vi "Teleop.vi"(10 "Match Info":T1={"Autonomous Elapsed Seconds"=0.0, "TeleOp Elapsed Seconds"=0.0, "Disabled Elapsed Seconds"=0.0, "Visited Autonomous"=FALSE, "Visited TeleOp"=FALSE, "Visited Disabled"=FALSE, "Autonomous Settings"={"Autonomous Style"=enum."Independent", "VI Refnum"=refnum}}, 11 "Call Context":T2) -> ()   [LabVIEW 2012]
doc: "This VI is called for each TeleOp packet received from the DS where the robot is not disabled. It is often used to read from the joysticks and update I/O or to update setpoints for timed control loops. It should complete and return within 20 milliseconds or it may miss DS packets."
uses:
  <vilib>/Rock Robotics/WPI/DriverStation/WPI_DriverStationDerivedRobotMode.ctl
  <vilib>/Rock Robotics/WPI/DriverStation/WPI_DriverStationMatch Info.ctl
  <vilib>/Rock Robotics/WPI/Joystick/WPI_JoystickAxis.ctl
  <vilib>/Rock Robotics/WPI/DriverStation/DriverStationLCD/WPI_DriverStationLCDLCDLine.ctl
  <vilib>/Rock Robotics/WPI/Solenoid/WPI_SolenoidValue.ctl
  Robot Global Data.vi
  <vilib>/Rock Robotics/WPI/Joystick/WPI_JoystickGetSetRefNum.vi
  <vilib>/Rock Robotics/WPI/RobotDrive/WPI_RobotDriveGetSetRefNum.vi
  <vilib>/Rock Robotics/WPI/Solenoid/WPI_SolenoidSetEnum.vi
panel:
  in  "ShifterState":bool
  in  "LifterState":bool
  out "Numeric 1":dbl(slide) scale=0.0..100.0
  out "Boolean 2":bool
  out "Boolean 1":bool
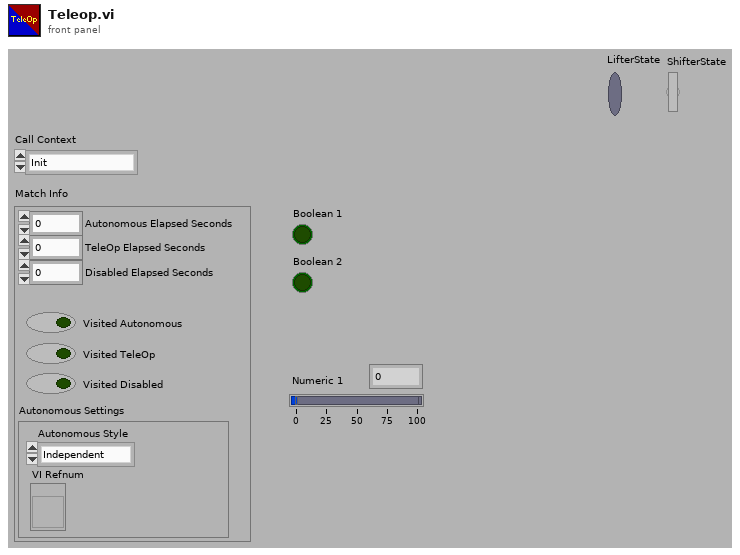
[diagram p1: front panel]
types:
  T1 = typedef "WPI_DriverStationMatch Info.ctl" = cluster{"Autonomous Elapsed Seconds":dbl, "TeleOp Elapsed Seconds":dbl, "Disabled Elapsed Seconds":dbl, "Visited Autonomous":bool, "Visited TeleOp":bool, "Visited Disabled":bool, "Autonomous Settings":cluster{"Autonomous Style":enum16{"Iterative", "Independent"}, "VI Refnum":refnum<vi>}}
  T2 = typedef "WPI_DriverStationDerivedRobotMode.ctl" = enum16{"Init", "Execute", "Stop"}
  T3 = typedef "WPI_JoystickAxis.ctl" = enum16{"Axis 1", "Axis 2", "Axis 3", "Axis 4", "Axis 5", "Axis 6"}
  T4 = typedef "WPI_JoystickDevRef.ctl" = cluster{"Device":T5}
  T5 = typedef "WPI_JoystickDeviceEnum.ctl" = enum16{"USB 1", "USB 2", "USB 3", "USB 4", "Kinect 1", "Kinect 2"}
  T6 = typedef "WPI_JoystickButtonState.ctl" = cluster{"Button 1":bool, "Button 2":bool, "Button 3":bool, "Button 4":bool, "Button 5":bool, "Button 6":bool, "Button 7":bool, "Button 8":bool, "Button 9":bool, "Button 10":bool, "Button 11":bool, "Button 12":bool}
  T7 = cluster{"axis 1 (x)":dbl, "axis 2 (y)":dbl, "axis 3 (throttle)":dbl, "axis 4":dbl, "axis 5":dbl, "axis 6":dbl}
  T8 = typedef "WPI_DriverStationLCDLCDLine.ctl" = enum16{"Main - Line 1", "User - Line 2", "User - Line 3", "User - Line 4", "User - Line 5", "User - Line 6"}
  T9 = typedef "WPI_SolenoidValue.ctl" = enum16{"Off", "On", "Forward", "Reverse"}
  T10 = typedef "WPI_MotorControlDeviceRef.ctl" = cluster{"DeviceStatus":errorcluster, "Type":enum16{"PWM", "CAN"}, "PWM":cluster{"Digital Module":T11, "PWM Channel":T12, "DeadBand":T13}, "CAN":cluster{"Device Number":u8, "Control Mode":T14, "Semaphore":T15, "Max Vout":dbl}, "Invert":bool, "TransformRef":T16, "InvTransformRef":T16}
  T11 = typedef "FPGA_TypedefDigitalModule.ctl" = enum16{"Digital Module 1", "Digital Module 2"}
  T12 = typedef "FPGA_DIOPWMChannel.ctl" = enum8{"PWM 1", "PWM 2", "PWM 3", "PWM 4", "PWM 5", "PWM 6", "PWM 7", "PWM 8", "PWM 9", "PWM 10", "Invalid"}
  T13 = typedef "WPI_PWMDeadband.ctl" = cluster{"Name":string, "maxPositivePwm":i32, "minPositivePwm":i32, "centerPwm":i32, "maxNegativePwm":i32, "minNegativePwm":i32, "angularRange":u16}
  T14 = typedef "WPI_CANJaguar_ControlMode.ctl" = enum8{"Percent VBus", "Current", "Speed", "Position", "Voltage"}
  T15 = typedef "Semaphore RefNum" = refnum<k1>
  T16 = typedef "WPI_PWMTransform_ConPane.ctl" = refnum<vi>
  T17 = typedef "WPI_SolenoidDevRef.ctl" = cluster{"DevStatus":errorcluster, "Solenoid Module":T18, "Forward Solenoid Channel":T19, "Reverse Solenoid Channel":T19}
  T18 = typedef "FPGA_TypedefSolenoidModule.ctl" = enum16{"Solenoid Module 1", "Solenoid Module 2"}
  T19 = typedef "WPI_SolenoidChannel.ctl" = enum8{"Solenoid 1", "Solenoid 2", "Solenoid 3", "Solenoid 4", "Solenoid 5", "Solenoid 6", "Solenoid 7", "Solenoid 8", "Invalid"}
  T20 = typedef "WPI_RobotDriveDevRef.ctl" = cluster{"DevStatus":errorcluster, "Motors[]":T10[], "Square Inputs":bool, "Max Output":dbl, "Isochronous":bool}
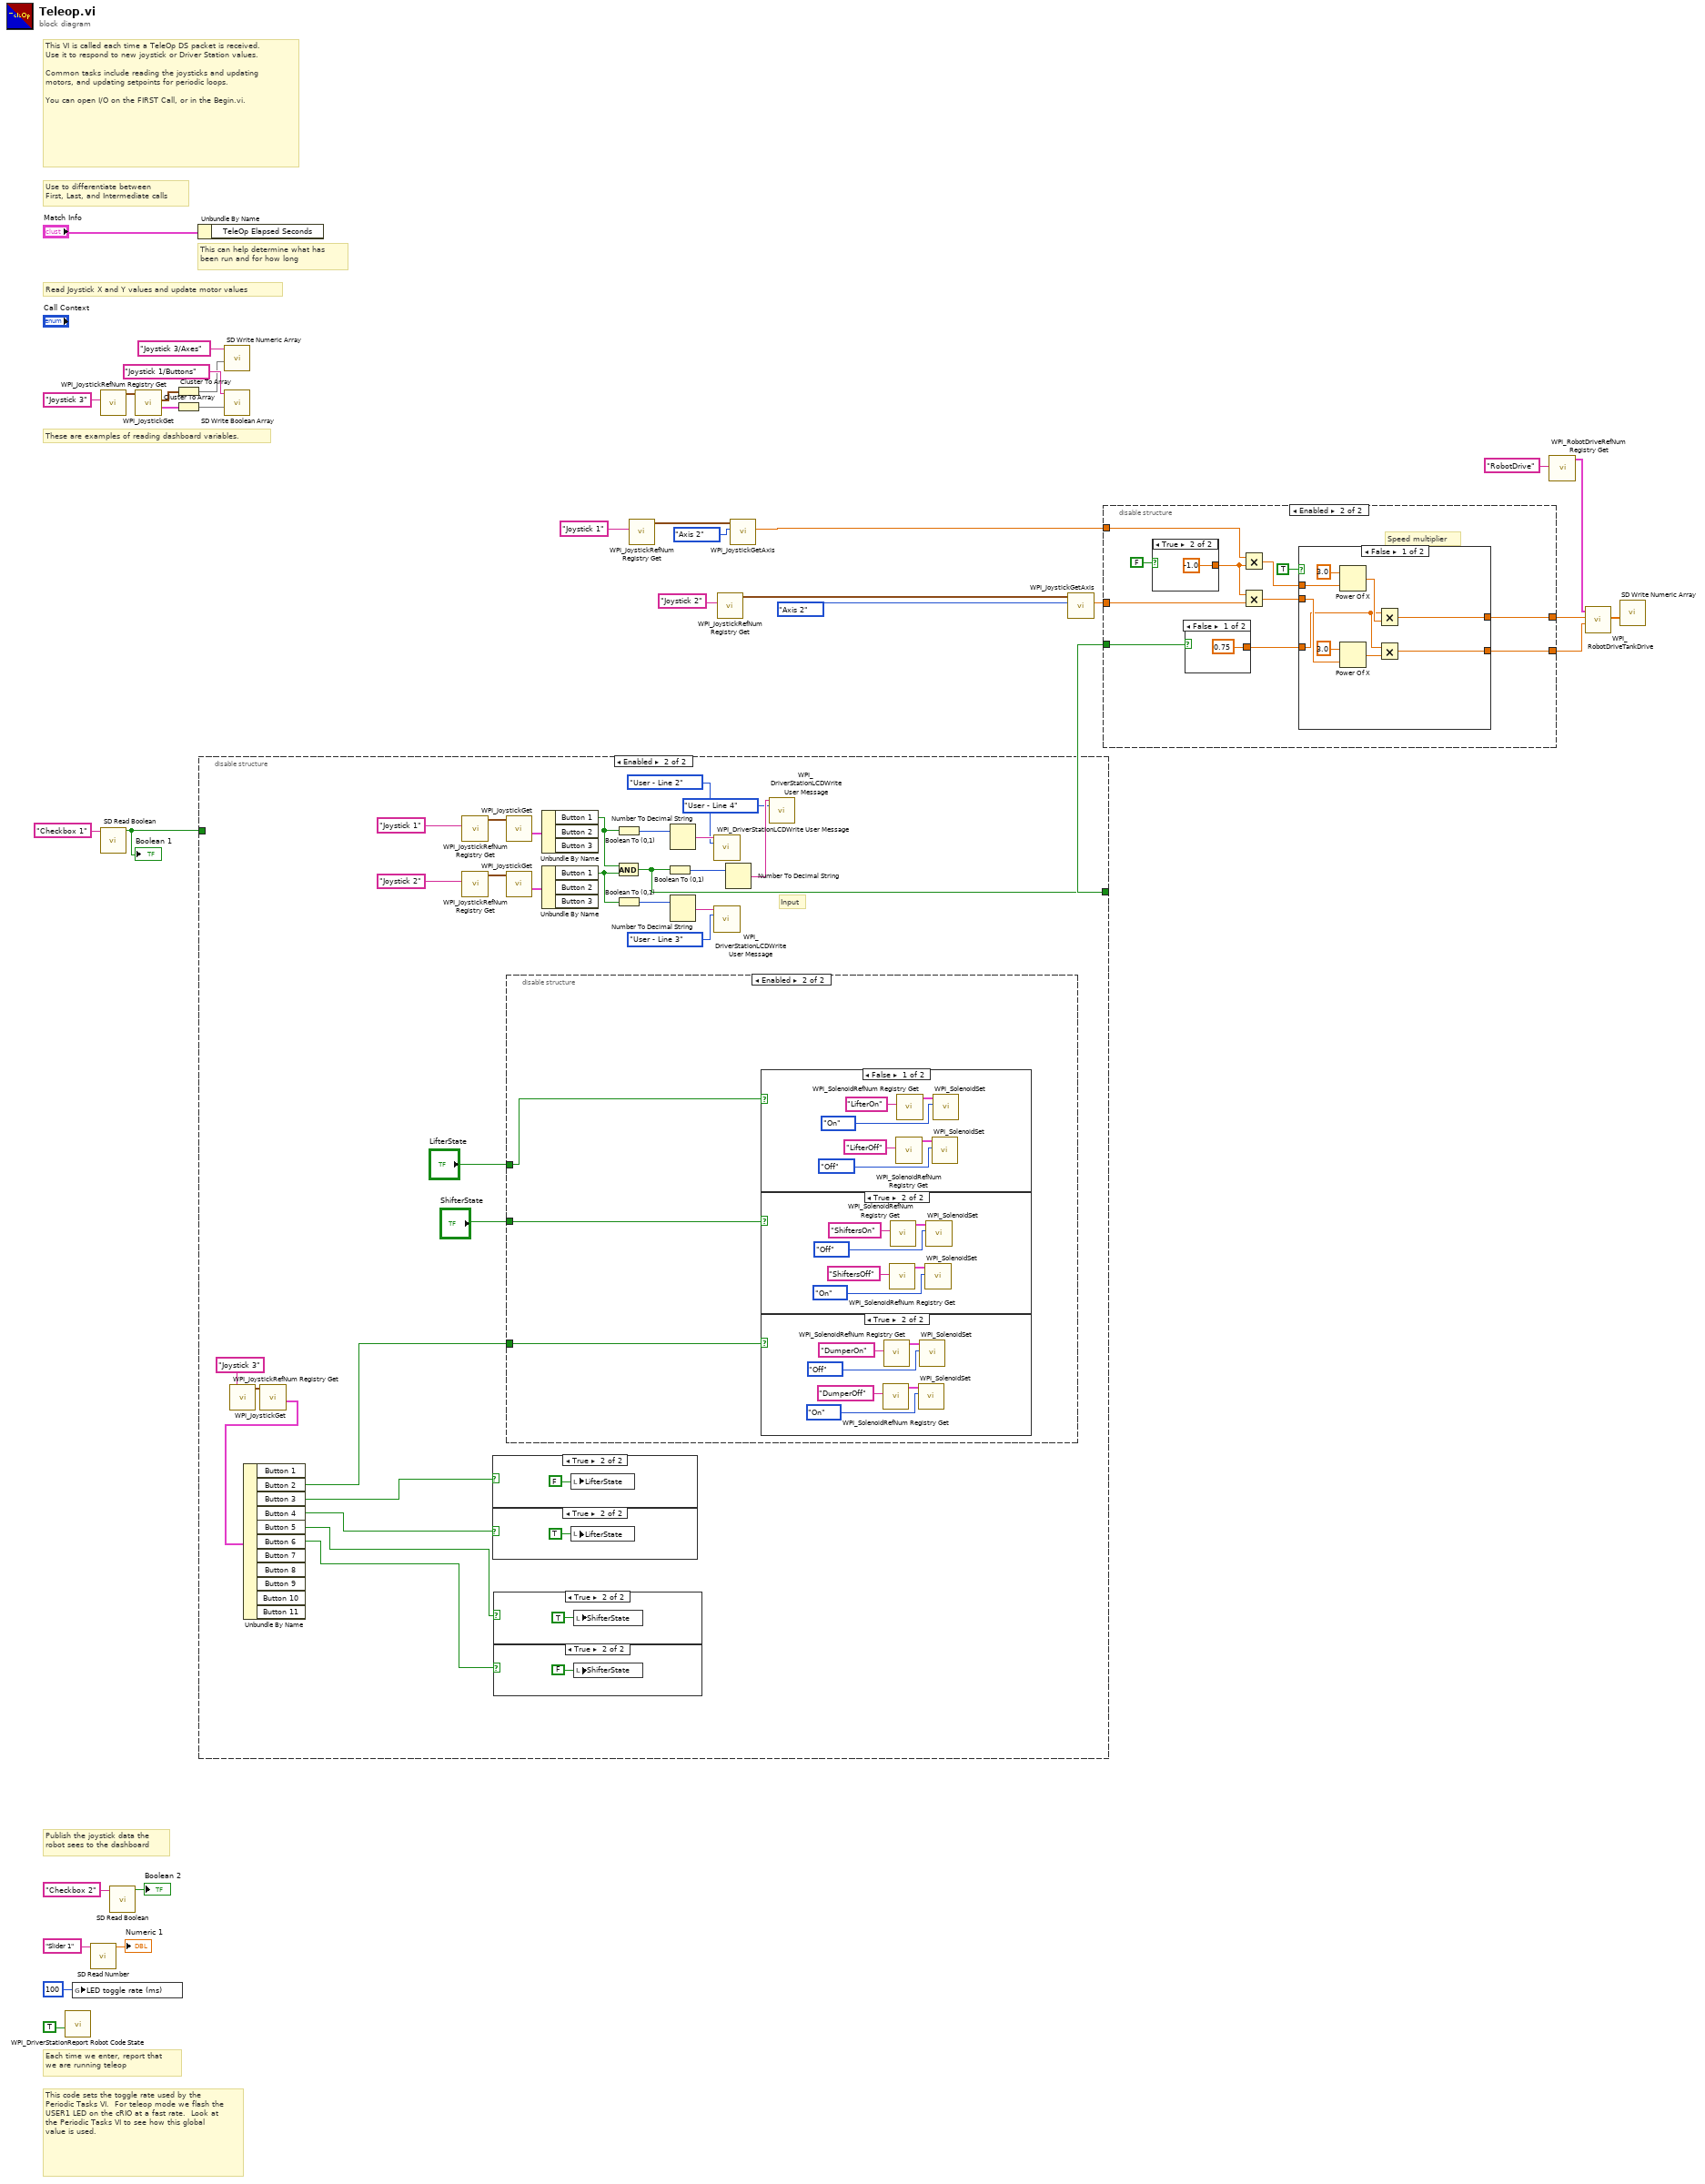
[diagram p0: block diagram]
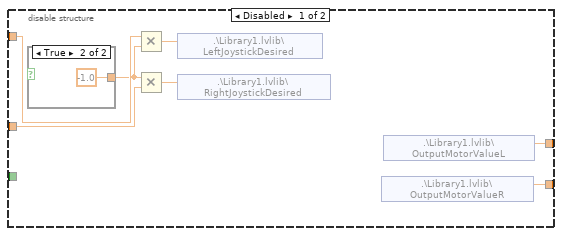
[diagram p2: hidden frame]
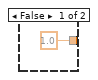
[diagram p3: hidden frame]
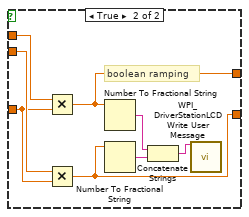
[diagram p4: hidden frame]
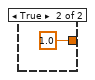
[diagram p5: hidden frame]
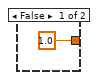
[diagram p6: hidden frame]
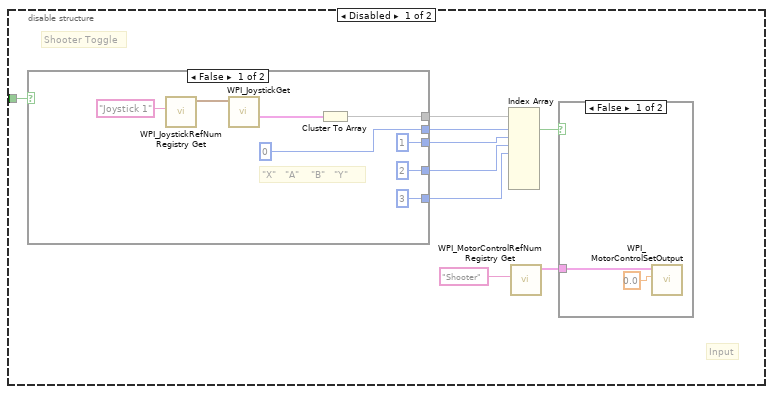
[diagram p7: hidden frame]
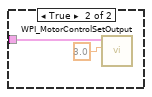
[diagram p8: hidden frame]
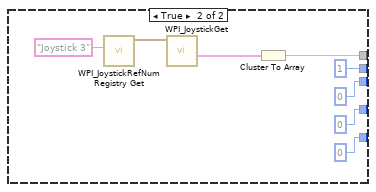
[diagram p9: hidden frame]
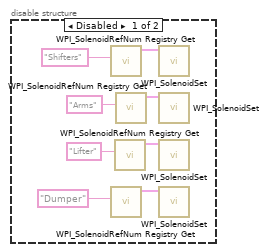
[diagram p14: hidden frame]
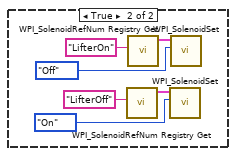
[diagram p15: hidden frame]
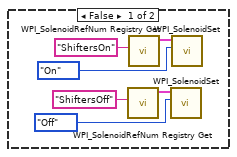
[diagram p16: hidden frame]
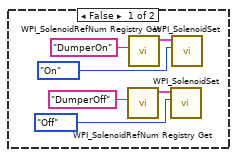
[diagram p17: hidden frame]
diagram:
  # "This code sets the toggle rate used by the Periodic Tasks VI.  For teleop mode we flash the USER1 LED on the cRIO at a fast rate.  Look at the Periodic Tasks VI to see how this global value is used."
  # "This VI is called each time a TeleOp DS packet is received.  Use it to respond to new joystick or Driver Station values.\n\nCommon tasks include reading the joysticks and updating motors, and updating setpoints for periodic loops.\n\nYou can open I/O on the FIRST Call, or in the Begin.vi."
  # "Publish the joystick data the\nrobot sees to the dashboard"
  # "These are examples of reading dashboard variables."
  # "Each time we enter, report that\nwe are running teleop"
  # "Use to differentiate between\nFirst, Last, and Intermediate calls"
  # "This can help determine what has\nbeen run and for how long"
  # "Read Joystick X and Y values and update motor values"
  n1 = call <vilib>:"WPI_DriverStationReport Robot Code State.vi"("TeleOp"=TRUE ("Autonomous")) -> ()  [unwired: 10 in, 1 out]
  n2 = global write "Robot Global Data.vi" "LED toggle rate (ms)"(u32 100 ("LED ms toggle rate")) -> ()
  n3 = call <vilib>:"SD Read Number.vi"("Name"="Slider 1" ("refnum name")) -> ("Numeric"=→"Numeric 1":dbl)  [unwired: 8 in, 2 out]
  n4 = call <vilib>:"WPI_JoystickRefNum Registry Get.vi"("refnum name"="Joystick 3") -> ("JoystickDevRef"=w22:T4)  [unwired: 1 in, 9 out]
  n5 = call <vilib>:"SD Read Boolean.vi"("Name"="Checkbox 1" ("refnum name")) -> ("Boolean"=w9:bool)  [unwired: 8 in, 2 out]
  "Boolean 1" <- w9
  n6 = call <vilib>:"SD Read Boolean.vi"("Name"="Checkbox 2" ("refnum name")) -> ("Boolean"=→"Boolean 2":bool)  [unwired: 8 in, 2 out]
  n7 = call <vilib>:"WPI_JoystickGet.vi"("JoystickDevRef"=w22) -> ("Buttons"=w21:T6, "Axes"=w18:T7)  [unwired: 1 in, 4 out]
  n8 = Cluster To Array(cluster=w18) -> (array=w20:dbl[])
  n9 = Cluster To Array(cluster=w21) -> (array=w25:bool[])
  n10 = Unbundle By Name("Match Info") -> ()  [unwired: 1 out]
  n11 = disable-structure shown="Enabled" {
    disable-tunnel: w9 -> [w40 _]
    disable-tunnel: [_ w74] -> w2
    frame Disabled {
      # "Input"
      # "Shooter Toggle"
      n12 = case shown="False" w40 {
        tunnel: [0 ("index") 1 ("index")] -> w39
        tunnel: [1 ("index") 0 ("index")] -> w34
        tunnel: [2 ("index") 0 ("index")] -> w36
        tunnel: [3 ("index") 0 ("index")] -> w35
        tunnel: [w48 w60] -> w37
        frame False {
          # "\"X\"   \"A\"    \"B\"   \"Y\""
          n13 = call <vilib>:"WPI_JoystickRefNum Registry Get.vi"("refnum name"="Joystick 1") -> ("JoystickDevRef"=w46:T4)  [unwired: 9 in, 1 out]
          n14 = call <vilib>:"WPI_JoystickGet.vi"("JoystickDevRef"=w46) -> ("Buttons"=w47:T6)  [unwired: 4 in, 2 out]
          n15 = Cluster To Array(cluster=w47) -> (array=w48:bool[])
        }
        frame True {
          n16 = call <vilib>:"WPI_JoystickRefNum Registry Get.vi"("refnum name"="Joystick 3") -> ("JoystickDevRef"=w58:T4)  [unwired: 9 in, 1 out]
          n17 = call <vilib>:"WPI_JoystickGet.vi"("JoystickDevRef"=w58) -> ("Buttons"=w59:T6)  [unwired: 4 in, 2 out]
          n18 = Cluster To Array(cluster=w59) -> (array=w60:bool[])
        }
      }
      n19 = Index Array(array=w37, index #1=w39, index #2=w34, index #3=w36, index #4=w35) -> (element #1=w38:bool)  [unwired: 4 in, 7 out]
      n20 = call <vilib>:"WPI_MotorControlRefNum Registry Get.vi"("refnum name"="Shooter") -> ("MotorControlDevRef"=w33:T10)  [unwired: 9 in, 1 out]
      n21 = case shown="False" w38 {
        tunnel: w33 -> [w42 w44]
        frame False {
          n22 = call <vilib>:"WPI_MotorControlSetOutput.vi"("Output"=0.0, "MotorControlDevRef"=w42) -> ()  [unwired: 7 in, 3 out]
        }
        frame True {
          n23 = call <vilib>:"WPI_MotorControlSetOutput.vi"("Output"=3.0, "MotorControlDevRef"=w44) -> ()  [unwired: 7 in, 3 out]
        }
      }
    }
    frame Enabled {
      # "Input"
      n24 = call <vilib>:"WPI_JoystickRefNum Registry Get.vi"("refnum name"="Joystick 3") -> ("JoystickDevRef"=w86:T4)  [unwired: 9 in, 1 out]
      n25 = call <vilib>:"WPI_JoystickGet.vi"("JoystickDevRef"=w86) -> ("Buttons"=w81:T6)  [unwired: 4 in, 2 out]
      n26 = Unbundle By Name(w81) -> ("Button 2"=w65:bool, "Button 3"=w64:bool, "Button 4"=w63:bool, "Button 5"=w62:bool, "Button 6"=w61:bool)  [unwired: 6 out]
      n27 = call <vilib>:"WPI_JoystickRefNum Registry Get.vi"("refnum name"="Joystick 1") -> ("JoystickDevRef"=w84:T4)  [unwired: 9 in, 1 out]
      n28 = call <vilib>:"WPI_JoystickRefNum Registry Get.vi"("refnum name"="Joystick 2") -> ("JoystickDevRef"=w80:T4)  [unwired: 9 in, 1 out]
      n29 = case shown="True" w64 {
        frame False {
        }
        frame True {
          n30 = local write "LifterState"(FALSE ("ArmState")) -> ()
        }
      }
      n31 = case shown="True" w63 {
        frame False {
        }
        frame True {
          n32 = local write "LifterState"(TRUE ("ArmState")) -> ()
        }
      }
      n33 = case shown="True" w62 {
        frame False {
        }
        frame True {
          n34 = local write "ShifterState"(TRUE ("ArmState")) -> ()
        }
      }
      n35 = case shown="True" w61 {
        frame False {
        }
        frame True {
          n36 = local write "ShifterState"(FALSE ("ArmState")) -> ()
        }
      }
      n37 = call <vilib>:"WPI_JoystickGet.vi"("JoystickDevRef"=w84) -> ("Buttons"=w82:T6)  [unwired: 4 in, 2 out]
      n38 = call <vilib>:"WPI_JoystickGet.vi"("JoystickDevRef"=w80) -> ("Buttons"=w78:T6)  [unwired: 4 in, 2 out]
      n39 = disable-structure shown="Enabled" {
        disable-tunnel: "LifterState" -> [_ w102]
        disable-tunnel: "ShifterState" -> [_ w103]
        disable-tunnel: w65 -> [_ w101]
        frame Disabled {
          n40 = call <vilib>:"WPI_SolenoidRefNum Registry Get.vi"("refnum name"="Shifters") -> ("SolenoidDevRef"=w99:T17)  [unwired: 9 in, 1 out]
          n41 = call <vilib>:"WPI_SolenoidRefNum Registry Get.vi"("refnum name"="Dumper") -> ("SolenoidDevRef"=w94:T17)  [unwired: 9 in, 1 out]
          n42 = call <vilib>:"WPI_SolenoidRefNum Registry Get.vi"("refnum name"="Lifter") -> ("SolenoidDevRef"=w98:T17)  [unwired: 9 in, 1 out]
          n43 = call <vilib>:"WPI_SolenoidRefNum Registry Get.vi"("refnum name"="Arms") -> ("SolenoidDevRef"=w96:T17)  [unwired: 9 in, 1 out]
          n44 = call-poly <vilib>:"WPI_SolenoidSet.vi"("SolenoidDevRef"=w99) -> ()  [unwired: 9 in, 2 out]
          n45 = call-poly <vilib>:"WPI_SolenoidSet.vi"("SolenoidDevRef"=w96) -> ()  [unwired: 9 in, 2 out]
          n46 = call-poly <vilib>:"WPI_SolenoidSet.vi"("SolenoidDevRef"=w98) -> ()  [unwired: 9 in, 2 out]
          n47 = call-poly <vilib>:"WPI_SolenoidSet.vi"("SolenoidDevRef"=w94) -> ()  [unwired: 9 in, 2 out]
        }
        frame Enabled {
          n48 = case shown="False" w102 {
            frame False {
              n49 = call <vilib>:"WPI_SolenoidRefNum Registry Get.vi"("refnum name"="LifterOff") -> ("SolenoidDevRef"=w106:T17)  [unwired: 9 in, 1 out]
              n50 = call <vilib>:"WPI_SolenoidRefNum Registry Get.vi"("refnum name"="LifterOn") -> ("SolenoidDevRef"=w108:T17)  [unwired: 9 in, 1 out]
              n51 = call-poly <vilib>:"WPI_SolenoidSet.vi"("Value"=WPI_SolenoidValue."Off", "SolenoidDevRef"=w106) -> ()  [unwired: 8 in, 2 out]
              n52 = call-poly <vilib>:"WPI_SolenoidSet.vi"("Value"=WPI_SolenoidValue."On", "SolenoidDevRef"=w108) -> ()  [unwired: 8 in, 2 out]
            }
            frame True {
              n53 = call <vilib>:"WPI_SolenoidRefNum Registry Get.vi"("refnum name"="LifterOff") -> ("SolenoidDevRef"=w112:T17)  [unwired: 9 in, 1 out]
              n54 = call <vilib>:"WPI_SolenoidRefNum Registry Get.vi"("refnum name"="LifterOn") -> ("SolenoidDevRef"=w114:T17)  [unwired: 9 in, 1 out]
              n55 = call-poly <vilib>:"WPI_SolenoidSet.vi"("Value"=WPI_SolenoidValue."On", "SolenoidDevRef"=w112) -> ()  [unwired: 8 in, 2 out]
              n56 = call-poly <vilib>:"WPI_SolenoidSet.vi"("Value"=WPI_SolenoidValue."Off", "SolenoidDevRef"=w114) -> ()  [unwired: 8 in, 2 out]
            }
          }
          n57 = case shown="True" w103 {
            frame False {
              n58 = call <vilib>:"WPI_SolenoidRefNum Registry Get.vi"("refnum name"="ShiftersOff") -> ("SolenoidDevRef"=w118:T17)  [unwired: 9 in, 1 out]
              n59 = call <vilib>:"WPI_SolenoidRefNum Registry Get.vi"("refnum name"="ShiftersOn") -> ("SolenoidDevRef"=w120:T17)  [unwired: 9 in, 1 out]
              n60 = call-poly <vilib>:"WPI_SolenoidSet.vi"("Value"=WPI_SolenoidValue."Off", "SolenoidDevRef"=w118) -> ()  [unwired: 8 in, 2 out]
              n61 = call-poly <vilib>:"WPI_SolenoidSet.vi"("Value"=WPI_SolenoidValue."On", "SolenoidDevRef"=w120) -> ()  [unwired: 8 in, 2 out]
            }
            frame True {
              n62 = call <vilib>:"WPI_SolenoidRefNum Registry Get.vi"("refnum name"="ShiftersOff") -> ("SolenoidDevRef"=w124:T17)  [unwired: 9 in, 1 out]
              n63 = call <vilib>:"WPI_SolenoidRefNum Registry Get.vi"("refnum name"="ShiftersOn") -> ("SolenoidDevRef"=w126:T17)  [unwired: 9 in, 1 out]
              n64 = call-poly <vilib>:"WPI_SolenoidSet.vi"("Value"=WPI_SolenoidValue."On", "SolenoidDevRef"=w124) -> ()  [unwired: 8 in, 2 out]
              n65 = call-poly <vilib>:"WPI_SolenoidSet.vi"("Value"=WPI_SolenoidValue."Off", "SolenoidDevRef"=w126) -> ()  [unwired: 8 in, 2 out]
            }
          }
          n66 = case shown="True" w101 {
            frame False {
              n67 = call <vilib>:"WPI_SolenoidRefNum Registry Get.vi"("refnum name"="DumperOff") -> ("SolenoidDevRef"=w130:T17)  [unwired: 9 in, 1 out]
              n68 = call <vilib>:"WPI_SolenoidRefNum Registry Get.vi"("refnum name"="DumperOn") -> ("SolenoidDevRef"=w132:T17)  [unwired: 9 in, 1 out]
              n69 = call-poly <vilib>:"WPI_SolenoidSet.vi"("Value"=WPI_SolenoidValue."Off", "SolenoidDevRef"=w130) -> ()  [unwired: 8 in, 2 out]
              n70 = call-poly <vilib>:"WPI_SolenoidSet.vi"("Value"=WPI_SolenoidValue."On", "SolenoidDevRef"=w132) -> ()  [unwired: 8 in, 2 out]
            }
            frame True {
              n71 = call <vilib>:"WPI_SolenoidRefNum Registry Get.vi"("refnum name"="DumperOff") -> ("SolenoidDevRef"=w136:T17)  [unwired: 9 in, 1 out]
              n72 = call <vilib>:"WPI_SolenoidRefNum Registry Get.vi"("refnum name"="DumperOn") -> ("SolenoidDevRef"=w138:T17)  [unwired: 9 in, 1 out]
              n73 = call-poly <vilib>:"WPI_SolenoidSet.vi"("Value"=WPI_SolenoidValue."On", "SolenoidDevRef"=w136) -> ()  [unwired: 8 in, 2 out]
              n74 = call-poly <vilib>:"WPI_SolenoidSet.vi"("Value"=WPI_SolenoidValue."Off", "SolenoidDevRef"=w138) -> ()  [unwired: 8 in, 2 out]
            }
          }
        }
      }
      n75 = Unbundle By Name(w82) -> ("Button 1"=w66:bool)  [unwired: 2 out]
      n76 = Unbundle By Name(w78) -> ("Button 1"=w70:bool)  [unwired: 2 out]
      n77 = Boolean To (0,1)(Boolean=w66) -> (0, 1=w69:i16)
      n78 = And(x=w66, y=w70) -> (x .and. y?=w74:bool)
      n79 = Boolean To (0,1)(Boolean=w70) -> (0, 1=w73:i16)
      n80 = Boolean To (0,1)(Boolean=w74) -> (0, 1=w77:i16)
      n81 = Number To Decimal String(number=w69) -> (decimal integer string=w68:string)  [unwired: 1 in]
      n82 = Number To Decimal String(number=w73) -> (decimal integer string=w72:string)  [unwired: 1 in]
      n83 = call <vilib>:"WPI_DriverStationLCDWrite User Message.vi"("line text"=w68, "line"=WPI_DriverStationLCDLCDLine."User - Line 2") -> ()  [unwired: 13 in, 1 out]
      n84 = call <vilib>:"WPI_DriverStationLCDWrite User Message.vi"("line text"=w72, "line"=WPI_DriverStationLCDLCDLine."User - Line 3") -> ()  [unwired: 13 in, 1 out]
      n85 = Number To Decimal String(number=w77) -> (decimal integer string=w76:string)  [unwired: 1 in]
      n86 = call <vilib>:"WPI_DriverStationLCDWrite User Message.vi"("line text"=w76, "line"=WPI_DriverStationLCDLCDLine."User - Line 4") -> ()  [unwired: 13 in, 1 out]
    }
  }
  n87 = call <vilib>:"SD Write Numeric Array.vi"("Numeric Array"=w20, "Name"="Joystick 3/Axes") -> ()  [unwired: 8 in, 2 out]
  n88 = call <vilib>:"SD Write Boolean Array.vi"("Boolean Array"=w25, "Name"="Joystick 1/Buttons") -> ()  [unwired: 8 in, 2 out]
  n89 = call <vilib>:"WPI_JoystickRefNum Registry Get.vi"("refnum name"="Joystick 1") -> ("JoystickDevRef"=w13:T4)  [unwired: 9 in, 1 out]
  n90 = call <vilib>:"WPI_JoystickRefNum Registry Get.vi"("refnum name"="Joystick 2") -> ("JoystickDevRef"=w11:T4)  [unwired: 9 in, 1 out]
  n91 = call <vilib>:"WPI_JoystickGetAxis.vi"("Axis"=WPI_JoystickAxis."Axis 2", "JoystickDevRef"=w13) -> ("Value"=w6:dbl)  [unwired: 8 in, 1 out]
  n92 = call <vilib>:"WPI_JoystickGetAxis.vi"("Axis"=WPI_JoystickAxis."Axis 2", "JoystickDevRef"=w11) -> ("Value"=w5:dbl)  [unwired: 8 in, 1 out]
  n93 = disable-structure shown="Enabled" {
    disable-tunnel: w6 -> [w146 w158]
    disable-tunnel: w5 -> [w144 w157]
    disable-tunnel: [w141 w152] -> w4
    disable-tunnel: [w140 w151] -> w3
    disable-tunnel: w2 -> [_ w154]
    frame Disabled {
      n94 = case shown="True" {
        selector: _ -> [_ _]
        tunnel: [1.0 ("y") -1.0 ("y")] -> w145
        frame False {
        }
        frame True {
        }
      }
      n95 = Multiply(x=w146, y=w145) -> (x*y=w143:dbl)
      n96 = Multiply(x=w145, y=w144) -> (x*y=w142:dbl)
      n97 = shared-variable ".\\Library1.lvlib\\LeftJoystickDesired"(w143) -> ()  [unwired: 1 in, 1 out]
      n98 = shared-variable ".\\Library1.lvlib\\RightJoystickDesired"(w142) -> ()  [unwired: 1 in, 1 out]
      n99 = shared-variable ".\\Library1.lvlib\\OutputMotorValueR"() -> (w140:dbl)  [unwired: 1 in, 1 out]
      n100 = shared-variable ".\\Library1.lvlib\\OutputMotorValueL"() -> (w141:dbl)  [unwired: 1 in, 1 out]
    }
    frame Enabled {
      # "Speed multiplier"
      n101 = case shown="True" FALSE {
        tunnel: [1.0 ("y") -1.0 ("y")] -> w159
        frame False {
        }
        frame True {
        }
      }
      n102 = case shown="False" w154 {
        tunnel: [0.75 ("y") 1.0 ("x")] -> w149
        frame False {
        }
        frame True {
        }
      }
      n103 = Multiply(x=w158, y=w159) -> (x*y=w156:dbl)
      n104 = Multiply(x=w159, y=w157) -> (x*y=w155:dbl)
      n105 = case shown="False" TRUE {
        tunnel: w156 -> [w168 w176]
        tunnel: w155 -> [w165 w175]
        tunnel: w149 -> [w162 w174]
        tunnel: [w160 w173] -> w152
        tunnel: [w161 w172] -> w151
        frame False {
          n106 = Power Of X(1:w168, 2:3.0 ("y")) -> (0:w164:dbl)
          n107 = Power Of X(1:w165, 2:3.0 ("y")) -> (0:w163:dbl)
          n108 = Multiply(x=w162, y=w164) -> (x*y=w160:dbl)
          n109 = Multiply(x=w162, y=w163) -> (x*y=w161:dbl)
        }
        frame True {
          # "boolean ramping"
          n110 = Multiply(x=w176, y=w174) -> (x*y=w173:dbl)
          n111 = Multiply(x=w175, y=w174) -> (x*y=w172:dbl)
          n112 = Number To Fractional String(number=w173) -> (F-format string=w170:string)  [unwired: 3 in]
          n113 = Number To Fractional String(number=w172) -> (F-format string=w169:string)  [unwired: 3 in]
          n114 = Concatenate Strings(w170, w169) -> (w171:string)
          n115 = call <vilib>:"WPI_DriverStationLCDWrite User Message.vi"("line text"=w171) -> ()  [unwired: 14 in, 1 out]
        }
      }
    }
  }
  n116 = call <vilib>:"WPI_RobotDriveRefNum Registry Get.vi"("refnum name"="RobotDrive") -> ("RobotDriveDevRef"=w15:T20)  [unwired: 1 in, 9 out]
  n117 = call <vilib>:"WPI_RobotDriveTankDrive.vi"("Right axis value"=w3, "Left axis value"=w4, "RobotDriveDevRef"=w15) -> ("Motor Values"=w10:dbl[])  [unwired: 6 in, 2 out]
  n118 = call <vilib>:"SD Write Numeric Array.vi"("Numeric Array"=w10) -> ()  [unwired: 9 in, 2 out]
